vi "GLOBALMain.vi"() -> ()   [LabVIEW 2011]
panel:
  out "Auton Files":string[](array[string])
  out "Number of Auton Files":dbl
  out "AutonArray":dbl[][](array[numeric])
  out "LED toggle rage (ms)":dbl
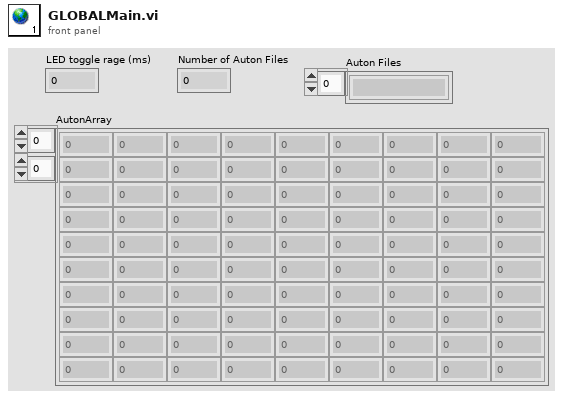
[diagram p1: front panel]
diagram:
